vi "formater n° cmde_V2.vi"(1 "NO_COMMANDE VAL":string, 2 "NO_COMMANDE LIV":string, 3 "NO_COMMANDE LIG":string, 4 "NO_COMMANDE":string) -> (0 "N° commande":string)   [LabVIEW 2020]
doc: "Formate les données NO_COMMANDE, NO_COMMANDE_LIV, NO_COMMANDE_LIG, NO_COMMANDE_VAL issues de la bdd pour mettre la commande au format habituel (ex: 6430/08-01.02.03)"
panel:
  # "Format BDD => INT"
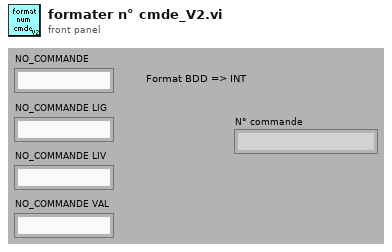
[diagram p1: front panel]
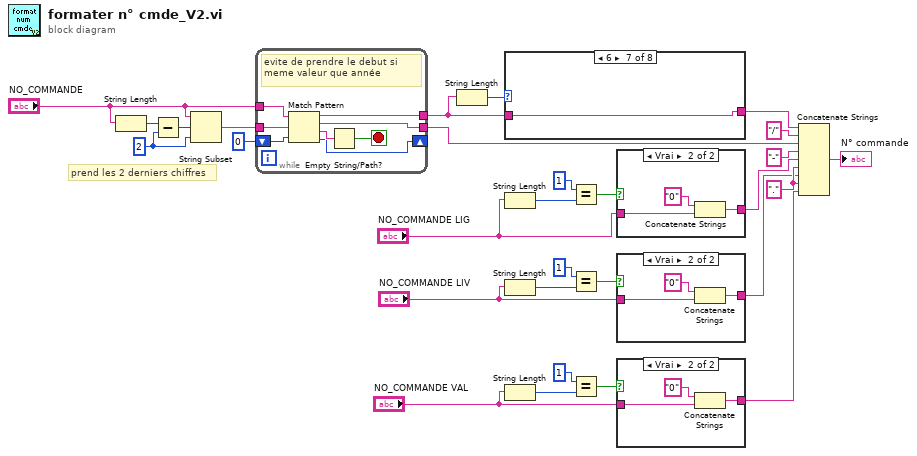
[diagram p0: block diagram]
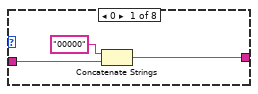
[diagram p5: hidden frame]
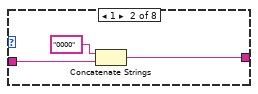
[diagram p6: hidden frame]
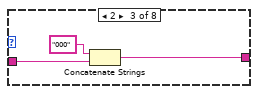
[diagram p7: hidden frame]
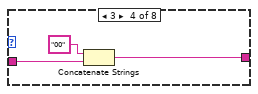
[diagram p8: hidden frame]
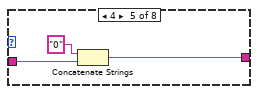
[diagram p9: hidden frame]
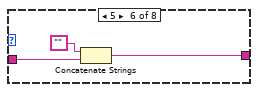
[diagram p10: hidden frame]
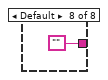
[diagram p11: hidden frame]
diagram:
  w10 = "."
  w27 = 2 ("y")
  # "prend les 2 derniers chiffres"
  n1 = String Length(string="NO_COMMANDE") -> (length=w29:i32)
  n2 = Subtract(x=w29, y=w27) -> (x-y=w28:i32)
  n3 = String Subset(string="NO_COMMANDE", offset (0)=w28, length (rest)=w27) -> (substring=w26:string)
  n4 = while {
    tunnel: [w35] -> w23
    tunnel: w26 -> [w37]
    tunnel: [w34] -> w8
    shift-right: [w30] -> _
    shift-left: 0 ("offset past match") -> [w31]
    tunnel: "NO_COMMANDE" -> [w36]
    stop <- w33 stop-if-true
    # "evite de prendre le debut si meme valeur que année"
    n5 = Match Pattern(string=w36, regular expression=w37, offset (0)=w31) -> (before substring=w35:string, match substring=w34:string, after substring=w32:string, offset past match=w30:i32)
    n6 = Empty String/Path?(string/path=w32) -> (empty?=w33:bool)
  }
  n7 = String Length(string=w23) -> (length=w24:i32)
  n8 = case shown="6" w24 {
    tunnel: w23 -> [w40 w42 w45 w48 w51 w54 w56 _]
    tunnel: [w38 w41 w44 w47 w50 w53 w56 ""] -> w9
    frame 0 {
      n9 = Concatenate Strings("00000" ("chaîne"), w40) -> (w38:string)
    }
    frame 1 {
      n10 = Concatenate Strings("0000" ("chaîne"), w42) -> (w41:string)
    }
    frame 2 {
      n11 = Concatenate Strings("000" ("chaîne"), w45) -> (w44:string)
    }
    frame 3 {
      n12 = Concatenate Strings("00" ("chaîne"), w48) -> (w47:string)
    }
    frame 4 {
      n13 = Concatenate Strings("0" ("chaîne"), w51) -> (w50:string)
    }
    frame 5 {
      n14 = Concatenate Strings("" ("chaîne"), w54) -> (w53:string)
    }
    frame 6 {
    }
    frame Default {
    }
  }
  n15 = String Length(string="NO_COMMANDE LIG") -> (length=w22:i32)
  n16 = String Length(string="NO_COMMANDE LIV") -> (length=w20:i32)
  n17 = String Length(string="NO_COMMANDE VAL") -> (length=w19:i32)
  n18 = Equal?(x=1 ("y"), y=w22) -> (x = y?=w18:bool)
  n19 = Equal?(x=1 ("y"), y=w20) -> (x = y?=w15:bool)
  n20 = Equal?(x=1 ("y"), y=w19) -> (x = y?=w16:bool)
  n21 = case shown="Vrai" w18 {
    tunnel: "NO_COMMANDE LIG" -> [w58 w60]
    tunnel: [w58 w59] -> w7
    frame False {
    }
    frame True {
      n22 = Concatenate Strings("0", w60) -> (w59:string)
    }
  }
  n23 = case shown="Vrai" w15 {
    tunnel: "NO_COMMANDE LIV" -> [w62 w64]
    tunnel: [w62 w63] -> w6
    frame False {
    }
    frame True {
      n24 = Concatenate Strings("0", w64) -> (w63:string)
    }
  }
  n25 = case shown="Vrai" w16 {
    tunnel: "NO_COMMANDE VAL" -> [w66 w68]
    tunnel: [w66 w67] -> w5
    frame False {
    }
    frame True {
      n26 = Concatenate Strings("0", w68) -> (w67:string)
    }
  }
  n27 = Concatenate Strings(w9, "/", w8, "-", w7, w10, w6, w10, w5) -> (→"N° commande":string)
